vi "Browse.vi"(6 "ns":u16=2, 8 "error in (no error)":errorcluster, 9 "id as String":string, 11 "Client In":refnum<class "Client.lvclass">) -> (0 "error out":errorcluster, 1 "result":T1[](array[typedef]), 2 "ret":i32, 3 "Client out":refnum<class "Client.lvclass">)   [LabVIEW 2017, in "opcua.lvlib" / "Client.lvclass"]
uses:
  Client.lvclass
  TypeDefs/Node.ctl
  Client.lvclass/Client.ctl
  opcua.lvlib
  opcua32.dll
panel:
  # "could be i=84\nor s=MyFolder"
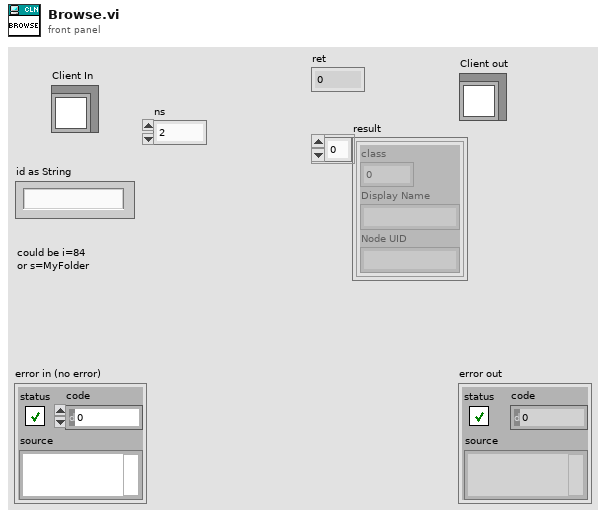
[diagram p1: front panel]
types:
  T1 = typedef "opcua.lvlib/Node.ctl" = cluster{"class":i32, "Display Name":string, "Node UID":string}
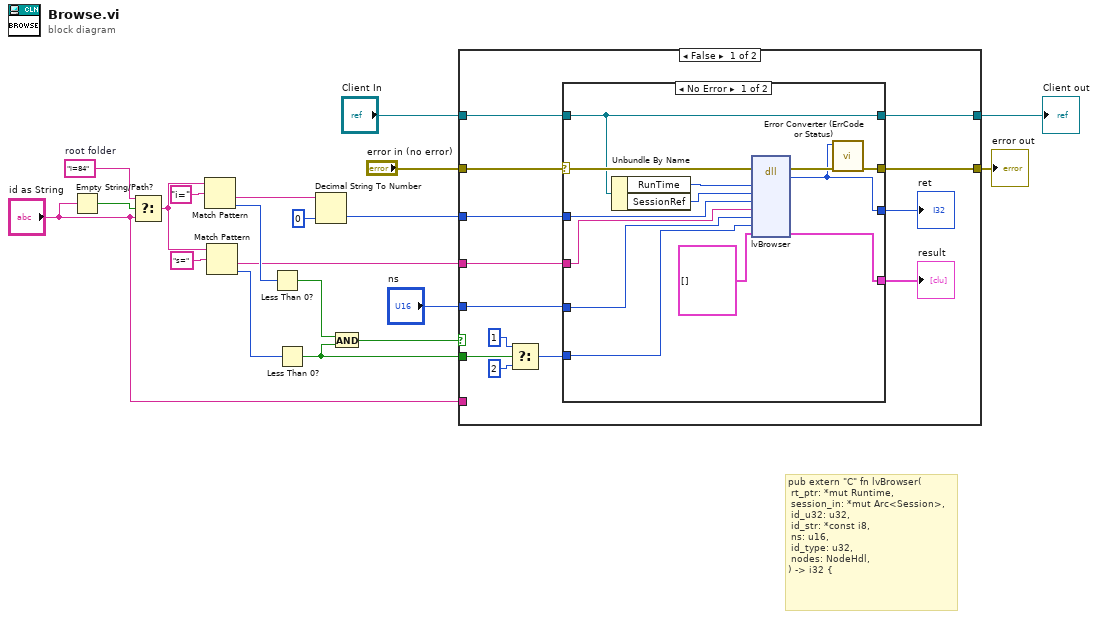
[diagram p0: block diagram]
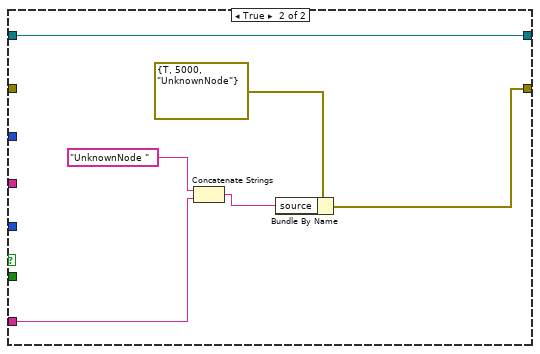
[diagram p3: hidden frame]
diagram:
  w3 = "i=84"  # root folder
  # "pub extern \"C\" fn lvBrowser(\n\trt_ptr: *mut Runtime,\n\tsession_in: *mut Arc<Session>,\n\tid_u32: u32,\n\tid_str: *const i8,\n\tns: u16,\n\tid_type: u32,\n\tnodes: NodeHdl,\n) -> i32 {"
  n1 = Empty String/Path?(string/path="id as String") -> (empty?=w4:bool)
  n2 = Select(t=w3, s=w4, f="id as String") -> (s? t:f=w2:string)
  n3 = Match Pattern(string=w2, regular expression="i=") -> (after substring=w12:string, offset past match=w11:i32)  [unwired: 1 in, 2 out]
  n4 = Match Pattern(string=w2, regular expression="s=") -> (after substring=w5:string, offset past match=w10:i32)  [unwired: 1 in, 2 out]
  n5 = Less Than 0?(x=w11) -> (x < 0?=w9:bool)
  n6 = Less Than 0?(x=w10) -> (x < 0?=w7:bool)
  n7 = Decimal String To Number(string=w12, default (0L)=u32 0 ("default (0 I32)")) -> (number=w14:u32)  [unwired: 1 in, 1 out]
  n8 = And(x=w9, y=w7) -> (x .and. y?=w8:bool)
  n9 = case shown="False" w8 {
    tunnel: "error in (no error)" -> [w33 _]
    tunnel: [w32 w49] -> w19
    tunnel: [w31 w54] -> w18
    tunnel: "Client In" -> [w30 w54]
    tunnel: w14 -> [w24 _]
    tunnel: w7 -> [w23 _]
    tunnel: w5 -> [w22 _]
    tunnel: "ns" -> [w21 _]
    tunnel: "id as String" -> [_ w51]
    frame False {
      n10 = Select(t=1, s=w23, f=2) -> (s? t:f=w25:i32)
      n11 = case shown="No Error" w33 {
        selector: w33 -> [w45 w47]
        tunnel: [w37 w47] -> w32
        tunnel: [w43 w48] -> w31
        tunnel: w30 -> [w43 w48]
        tunnel: [w36 _] -> w29
        tunnel: [w42 _] -> w28
        tunnel: w22 -> [w41 _]
        tunnel: w25 -> [w34 _]
        tunnel: w24 -> [w40 _]
        tunnel: w21 -> [w39 _]
        frame No Error {
          n12 = Unbundle By Name(w43) -> ("RunTime"=w44:u64, "SessionRef"=w46:u64)
          n13 = dll-call lib="C:/Users/Andrey/Desktop/opcua-labview/opcua-lvlib/opcua*.dll" fn="lvBrowser"(error in=w45, "RunTime"=w44, "session"=w46, "id"=w40, "str"=w41, "ns"=w39, "type"=w34, "result"=T1[] []) -> (error out=w38:errorcluster, "return type"=w36:i32, "result"=w42:T1[])  [unwired: 8 in, 1 out]
          n14 = call "Error Converter (ErrCode or Status).vi"("error in (no error)"=w38, "error code"=w36) -> ("error out"=w37:errorcluster)  [unwired: 9 in]
        }
        frame Error {
        }
      }
      "ret" <- w29
      "result" <- w28
    }
    frame True {
      n15 = Concatenate Strings("UnknownNode " ("source"), w51) -> (w50:string)
      n16 = Bundle By Name(cluster=errorcluster {"status"=TRUE, "code"=5000, "source"="UnknownNode"} ("error IO"), "source"=w50) -> (w49:errorcluster)
    }
  }
  "error out" <- w19
  "Client out" <- w18
